vi "obtainReferenceToAConditionalDisableStructure.vi"(8 "error in (no error)":errorcluster, 11 "VI in":refnum<class "VI.lvclass">) -> (0 "error out":errorcluster, 2 "Node Refnum CDS Source":refnum<vi>, 3 "VI out":refnum<class "VI.lvclass">)   [LabVIEW 2016, in "VI.lvclass"]
uses:
  VI.lvclass
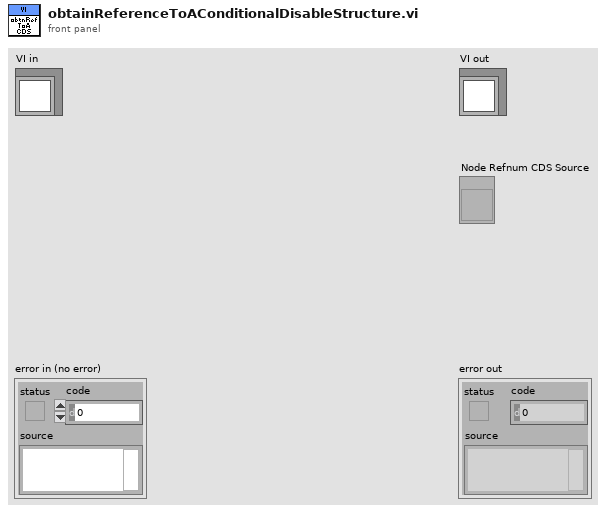
[diagram p1: front panel]
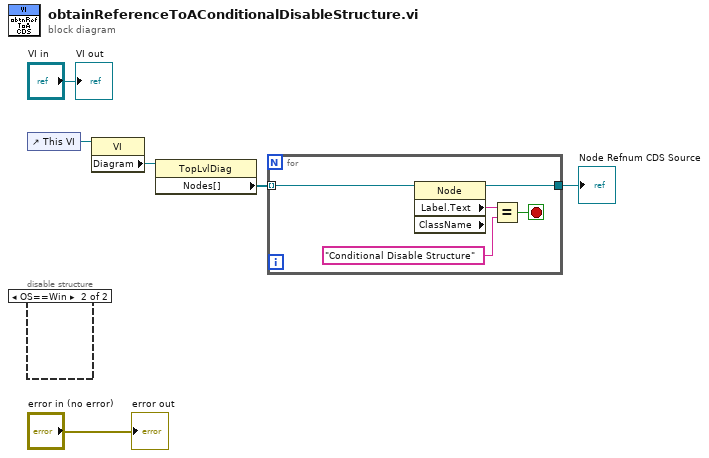
[diagram p0: block diagram]
diagram:
  n1 = control-ref of="This VI"() -> (w2:refnum<vi>)
  n2 = disable-structure "Conditional Disable Structure" shown="OS==Win" {
    frame condition #0 {
    }
    frame condition #1 (active) {
    }
  }
  n3 = property on="Property Node" class="VI"(reference=w2) -> ("Diagram"=w3:refnum<vi>)  [unwired: 1 in, 2 out]
  n4 = property on="Property Node" class="TopLvlDiag"(reference=w3) -> ("Nodes[]"=w4:refnum<vi>[])  [unwired: 1 in, 2 out]
  n5 = for {
    tunnel: w4 -> [w11] mode=indexing
    tunnel: [w8] -> w1
    stop <- w9 stop-if-true
    n6 = property class="Node" props=["Label", "Text", "ClassName"](reference=w11) -> (reference out=w8:refnum<vi>, "Label.Text"=w7:string)  [unwired: 1 in, 2 out]
    n7 = Equal?(x=w7, y="Conditional Disable Structure" ("Class Name")) -> (x = y?=w9:bool)
  }
  "Node Refnum CDS Source" <- w1
  "error out" <- "error in (no error)"
  "VI out" <- "VI in"
